vi "write_jt_scan_settings_to_data_file.vi"(10 "J-V-t Scan Settings":T1={"Bias 1"=20.0, "Bias 2 "=0.0, "t for bias 1 (s)"=60.0, "t for bias 2 (s)"=120.0, "Enable display"=0, "Electrode configuration"=1, "Bias 1 mode"=0, "Bias 2 mode"=0, "Current range for bias 1"=0, "Current range for bias 2"=0, "Voltage range for bias 1"=0, "Voltage range for bias 2"=0, "Settling delay (ms)"=1.0, "Auto settling delay"=1, "Integration time (ms)"=1.0} {"Integration time (ms)" min=0.2; "Auto settling delay" items=["False", "True"]; "Settling delay (ms)" min=0.0; "Voltage range for bias 2" items=["Auto", "200 mV", "2 V", "20 V", "200 V"]; "Voltage range for bias 1" items=["Auto", "200 mV", "2 V", "20 V", "200 V"]; "Current range for bias 2" items=["Auto", "1 uA", "10 uA", "100 uA", "1 mA", "10 mA", "100 mA", "1 A"]; "Current range for bias 1" items=["Auto", "1 uA", "10 uA", "100 uA", "1 mA", "10 mA", "100 mA", "1 A"]; "Bias 2 mode" items=["V", "A"]; "Bias 1 mode" items=["V", "A"]; "Electrode configuration" items=["2-wire", "4-wire"]; "Enable display" items=["False", "True"]; "t for bias 2 (s)" min=0.0; "t for bias 1 (s)" min=0.0}, 11 "file path in":path) -> (3 "file path out":path)   [LabVIEW 2016]
uses:
  TypeDefs/j-t_settings.ctl
  <vilib>/Utility/file.llb/Write Delimited Spreadsheet (string).vi
panel:
  out "Electrode configuration":u16(ring)=1 items=["2-wire", "4-wire"]
  out "Auto settling delay":u16(ring)=1 items=["False", "True"]
  out "Voltage range for bias 2":u16(ring) items=["Auto", "200 mV", "2 V", "20 V", "200 V"]
  out "Voltage range for bias 1":u16(ring) items=["Auto", "200 mV", "2 V", "20 V", "200 V"]
  out "Current range for bias 2":u16(ring) items=["Auto", "1 uA", "10 uA", "100 uA", "1 mA", "10 mA", "100 mA", "1 A"]
  out "Current range for bias 1":u16(ring) items=["Auto", "1 uA", "10 uA", "100 uA", "1 mA", "10 mA", "100 mA", "1 A"]
  out "Bias 2 mode":u16(ring) items=["V", "A"]
  out "Bias 1 mode":u16(ring) items=["V", "A"]
  out "scan settings":string[][](array[string])
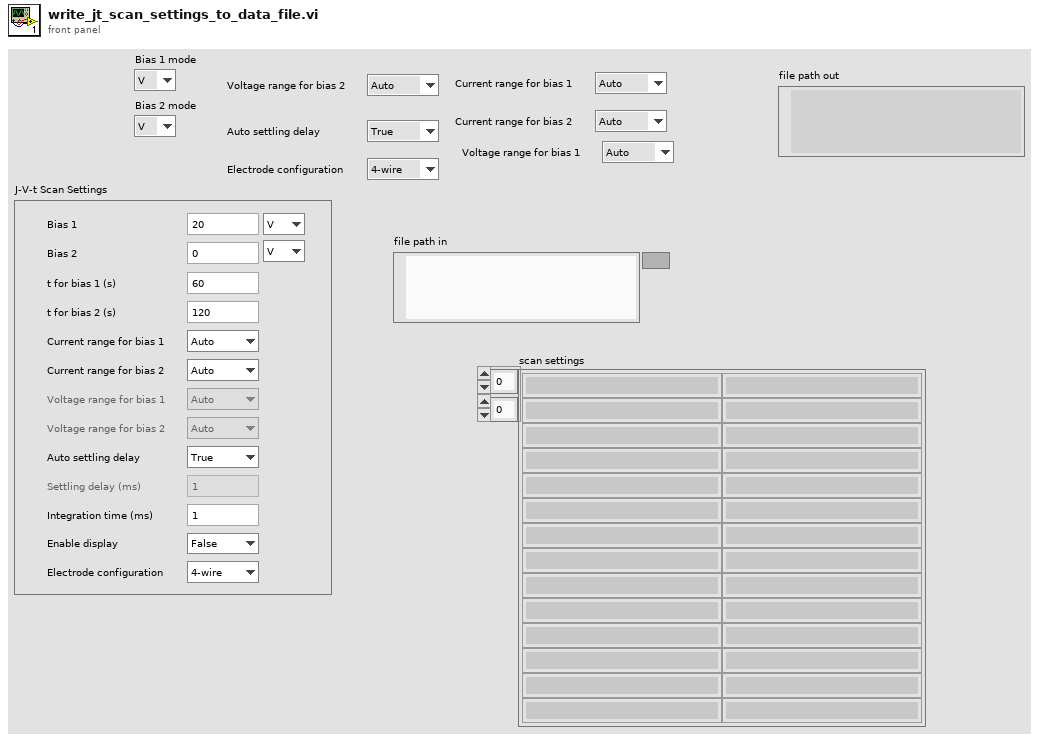
[diagram p1: front panel]
types:
  T1 = typedef "j-t_settings.ctl" = cluster{"Bias 1":dbl, "Bias 2 ":dbl, "t for bias 1 (s)":dbl, "t for bias 2 (s)":dbl, "Enable display":u16, "Electrode configuration":u16, "Bias 1 mode":u16, "Bias 2 mode":u16, "Current range for bias 1":u16, "Current range for bias 2":u16, "Voltage range for bias 1":u16, "Voltage range for bias 2":u16, "Settling delay (ms)":dbl, "Auto settling delay":u16, "Integration time (ms)":dbl}
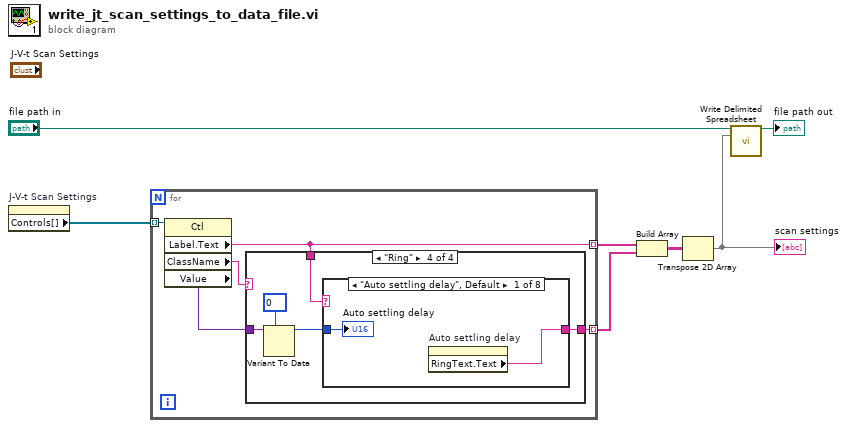
[diagram p0: block diagram]
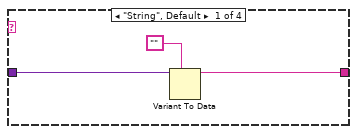
[diagram p2: hidden frame]
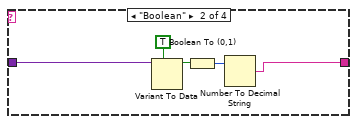
[diagram p3: hidden frame]
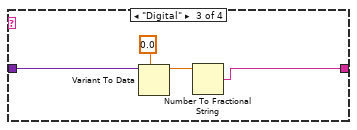
[diagram p4: hidden frame]
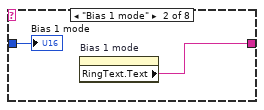
[diagram p5: hidden frame]
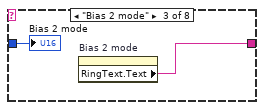
[diagram p6: hidden frame]
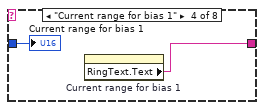
[diagram p7: hidden frame]
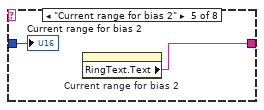
[diagram p8: hidden frame]
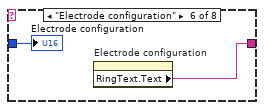
[diagram p9: hidden frame]
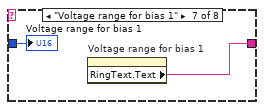
[diagram p10: hidden frame]
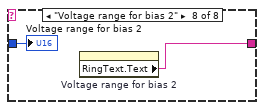
[diagram p11: hidden frame]
diagram:
  n1 = property on="J-V-t Scan Settings" class="Clust (strict)"() -> ("Controls[]"=w1:refnum<vi>[])  [unwired: 2 in, 2 out]
  n2 = for {
    tunnel: w1 -> [w12] mode=indexing
    tunnel: [w8] -> w7 mode=indexing
    tunnel: [w9] -> w5 mode=indexing
    n3 = property class="Ctl"(reference=w12) -> ("Label.Text"=w8:string, "ClassName"=w11:string, "Value"=w10:variant)  [unwired: 1 in, 2 out]
    n4 = case shown="\"Ring\"" w11 {
      tunnel: [w14 w17 w22 w26] -> w9
      tunnel: w10 -> [w13 w16 w21 w29]
      tunnel: w8 -> [_ _ _ w27]
      frame "String", Default {
        n5 = Variant To Data(type="", Variant=w13) -> (data=w14:string)  [unwired: 1 in, 1 out]
      }
      frame "Boolean" {
        n6 = Variant To Data(type=TRUE, Variant=w16) -> (data=w19:bool)  [unwired: 1 in, 1 out]
        n7 = Boolean To (0,1)(Boolean=w19) -> (0, 1=w18:i16)
        n8 = Number To Decimal String(number=w18) -> (decimal integer string=w17:string)  [unwired: 1 in]
      }
      frame "Digital" {
        n9 = Variant To Data(type=0.0, Variant=w21) -> (data=w23:dbl)  [unwired: 1 in, 1 out]
        n10 = Number To Fractional String(number=w23) -> (F-format string=w22:string)  [unwired: 3 in]
      }
      frame "Ring" {
        w28 = u16 0 items=[""]
        n11 = Variant To Data(type=w28, Variant=w29) -> (data=w25:u16)  [unwired: 1 in, 1 out]
        n12 = case shown="\"Auto settling delay\", Default" w27 {
          tunnel: [w30 w32 w34 w36 w38 w40 w42 w44] -> w26
          tunnel: w25 -> [w31 w33 w35 w37 w39 w41 w43 w45]
          frame "Auto settling delay", Default {
            n13 = property on="Auto settling delay" class="Ring (strict)"() -> ("RingText.Text"=w30:string)  [unwired: 2 in, 2 out]
            "Auto settling delay" <- w31
          }
          frame "Bias 1 mode" {
            n14 = property on="Bias 1 mode" class="Ring (strict)"() -> ("RingText.Text"=w32:string)  [unwired: 2 in, 2 out]
            "Bias 1 mode" <- w33
          }
          frame "Bias 2 mode" {
            n15 = property on="Bias 2 mode" class="Ring (strict)"() -> ("RingText.Text"=w34:string)  [unwired: 2 in, 2 out]
            "Bias 2 mode" <- w35
          }
          frame "Current range for bias 1" {
            n16 = property on="Current range for bias 1" class="Ring (strict)"() -> ("RingText.Text"=w36:string)  [unwired: 2 in, 2 out]
            "Current range for bias 1" <- w37
          }
          frame "Current range for bias 2" {
            n17 = property on="Current range for bias 2" class="Ring (strict)"() -> ("RingText.Text"=w38:string)  [unwired: 2 in, 2 out]
            "Current range for bias 2" <- w39
          }
          frame "Electrode configuration" {
            n18 = property on="Electrode configuration" class="Ring (strict)"() -> ("RingText.Text"=w40:string)  [unwired: 2 in, 2 out]
            "Electrode configuration" <- w41
          }
          frame "Voltage range for bias 1" {
            n19 = property on="Voltage range for bias 1" class="Ring (strict)"() -> ("RingText.Text"=w42:string)  [unwired: 2 in, 2 out]
            "Voltage range for bias 1" <- w43
          }
          frame "Voltage range for bias 2" {
            n20 = property on="Voltage range for bias 2" class="Ring (strict)"() -> ("RingText.Text"=w44:string)  [unwired: 2 in, 2 out]
            "Voltage range for bias 2" <- w45
          }
        }
      }
    }
  }
  n21 = Build Array(w7, w5) -> (w6:string[][])
  n22 = Transpose 2D Array(2D array=w6) -> (transposed array=w4:string[][])
  "scan settings" <- w4
  n23 = call-poly <vilib>:"Write Delimited Spreadsheet.vi"("file path (dialog if empty)"="file path in", "2D data"=w4) -> ("new file path (Not A Path if cancelled)"=→"file path out":path)  [unwired: 12 in, 1 out]
